vi "Write y.vi"(8 "error in (no error)":errorcluster, 10 "y":sgl, 11 "Vector2 in":refnum<class "Vector2.lvclass">) -> (0 "error out":errorcluster, 3 "Vector2 out":refnum<class "Vector2.lvclass">)   [LabVIEW 2022 SP3, in "Vector2.lvclass"]
uses:
  Vector2.lvclass
  Vector2.lvclass/Vector2.ctl
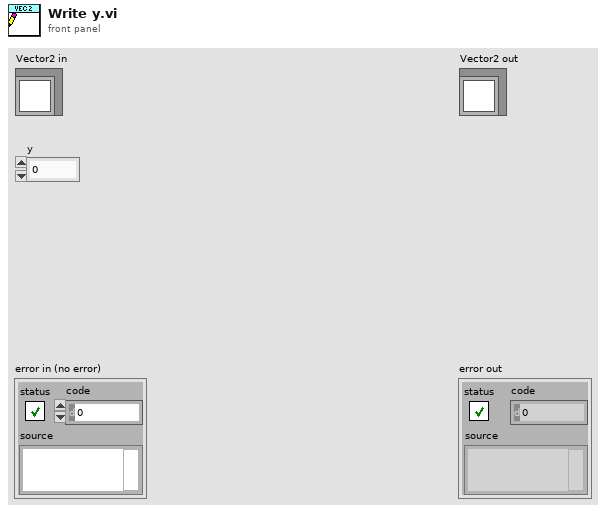
[diagram p1: front panel]
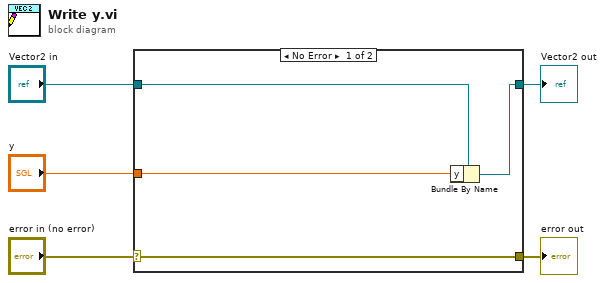
[diagram p0: block diagram]
diagram:
  n1 = case shown="No Error" "error in (no error)" {
    selector: "error in (no error)" -> [w9 w10]
    tunnel: [w9 w10] -> w4
    tunnel: [w7 w11] -> w2
    tunnel: "Vector2 in" -> [w8 w11]
    tunnel: "y" -> [w6 _]
    frame No Error {
      n2 = Bundle By Name(cluster=w8, "y"=w6) -> (w7:refnum<class "Vector2.lvclass">)
    }
    frame Error {
    }
  }
  "error out" <- w4
  "Vector2 out" <- w2
